vi "Read Run.vi"(8 "error in (no error)":errorcluster, 11 "SyncPluginBase in":refnum<class "SyncPluginBase.lvclass">) -> (0 "error out":errorcluster, 2 "Run":bool, 3 "SyncPluginBase out":refnum<class "SyncPluginBase.lvclass">)   [LabVIEW 2014, in "SyncPlugins.lvlib" / "SyncPluginBase.lvclass"]
uses:
  SyncPluginBase.lvclass
  SyncPluginBase.lvclass/SyncPluginBase.ctl
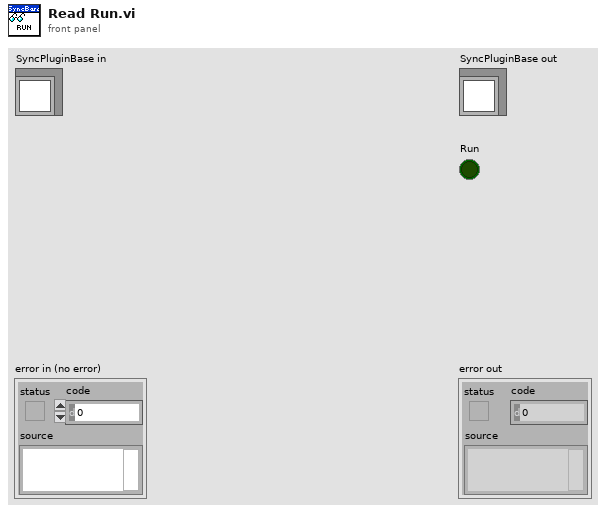
[diagram p1: front panel]
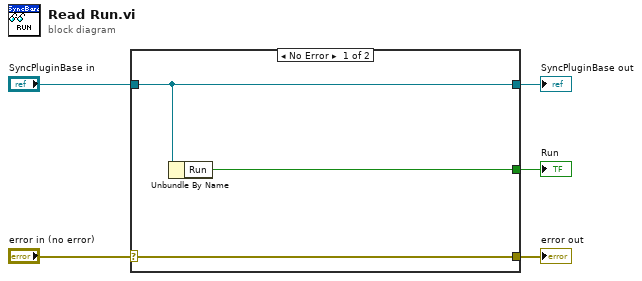
[diagram p0: block diagram]
diagram:
  n1 = case shown="No Error" "error in (no error)" {
    selector: "error in (no error)" -> [w8 w9]
    tunnel: [w8 w9] -> w4
    tunnel: [w7 w10] -> w2
    tunnel: "SyncPluginBase in" -> [w7 w10]
    tunnel: [w6 _] -> w1
    frame No Error {
      n2 = Unbundle By Name(w7) -> ("Run"=w6:bool)
    }
    frame Error {
    }
  }
  "error out" <- w4
  "SyncPluginBase out" <- w2
  "Run" <- w1
